vi "Library.GetMemberVIs.vi"(8 "error in (no error)":errorcluster, 11 "Library Reference":refnum<vi>) -> (0 "error out":errorcluster, 1 "Item Type":string[](array[string]), 2 "Member VI References":refnum<vi>[](array[refnum]), 3 "Library Reference (dup)":refnum<vi>)   [LabVIEW 2011]
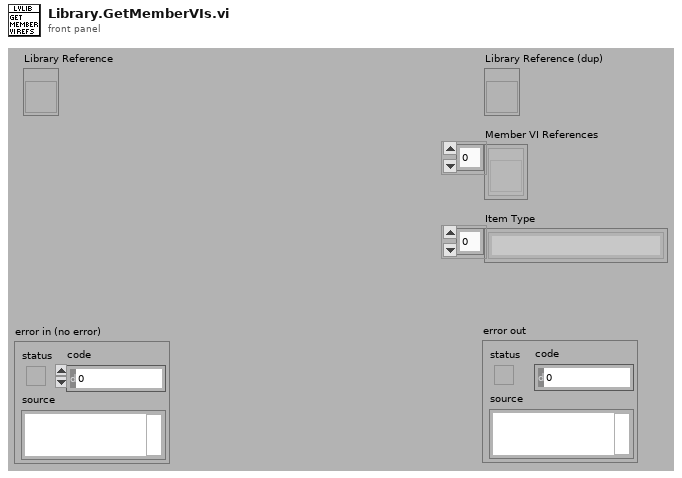
[diagram p1: front panel]
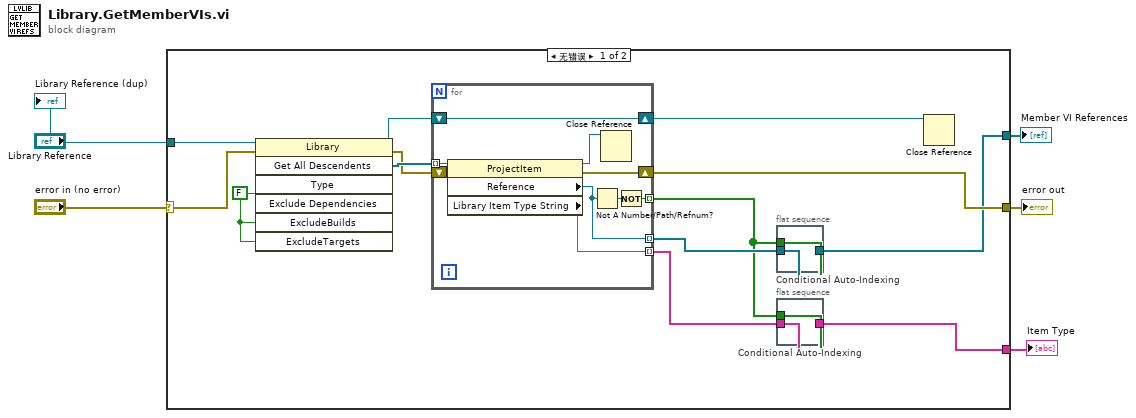
[diagram p0: block diagram]
diagram:
  n1 = case shown="无错误" "error in (no error)" {
    selector: "error in (no error)" -> [w13 w56]
    tunnel: [w10 _] -> w5
    tunnel: [w14 w56] -> w4
    tunnel: "Library Reference" -> [w6 _]
    tunnel: [w7 _] -> w1
    frame No Error {
      w12 = FALSE ("ExcludeDependencies")
      n2 = invoke class="Library" method="Get All Descendents"(reference=w6, error in=w13, "Exclude Dependencies"=w12, "ExcludeBuilds"=w12, "ExcludeTargets"=w12) -> (reference out=w16:refnum<vi>, error out=w17:errorcluster, "All Descendents"=w18:refnum<vi>[])  [unwired: 2 in, 4 out]
      n3 = for {
        tunnel: w18 -> [w55] mode=indexing
        tunnel: [w53] -> w9 mode=indexing
        tunnel: [w52] -> w11 mode=indexing
        shift-right: [w51] -> w14
        shift-left: w17 -> [w50]
        shift-right: [w48] -> w15
        shift-left: w16 -> [w48]
        tunnel: [w47] -> w8 mode=indexing
        n4 = property class="ProjectItem"(reference=w55, error in=w50) -> (reference out=w49:refnum<vi>, error out=w51:errorcluster, "Reference"=w52:refnum<vi>, "Library Item Type String"=w47:string)
        n5 = Not A Number/Path/Refnum?(number/path/refnum=w52) -> (NaN/Path/Refnum?=w54:bool)
        n6 = Close Reference(reference=w49) -> ()  [unwired: 1 in, 1 out]
        n7 = Not(x=w54) -> (.not. x?=w53:bool)
      }
      n8 = flat-sequence "Conditional Auto-Indexing" {
        tunnel: w9 -> [w35]
        tunnel: w11 -> [w34]
        tunnel: [w33] -> w10
        frame #0 {
          n9 = Boolean To (0,1)(Boolean=w35) -> (0, 1=w38:i16[])
          n10 = To Unsigned Long Integer(number=w38) -> (unsigned 32bit integer=w39:u32[])
          n11 = Add Array Elements(numeric array=w39) -> (sum=w37:u32)
          n12 = for {
            N: w37 -> [_]
            tunnel: w34 -> [w42]
            tunnel: w35 -> [w46]
            shift-right: [w43] -> _
            shift-left: -1 ("start index (0)") -> [w44]
            tunnel: [w41] -> w33 mode=indexing
            # "index out that element"
            # "Find the next element to keep"
            n13 = Increment(x=w44) -> (x+1=w40:i32)
            n14 = Search 1D Array(1D array=w46, element=TRUE, start index (0)=w40) -> (index of element=w43:i32)
            n15 = Index Array(array=w42, index=w43) -> (element=w41:refnum<vi>)
          }
        }
      }
      n16 = flat-sequence "Conditional Auto-Indexing" {
        tunnel: w9 -> [w21]
        tunnel: w8 -> [w20]
        tunnel: [w19] -> w7
        frame #0 {
          n17 = Boolean To (0,1)(Boolean=w21) -> (0, 1=w24:i16[])
          n18 = To Unsigned Long Integer(number=w24) -> (unsigned 32bit integer=w25:u32[])
          n19 = Add Array Elements(numeric array=w25) -> (sum=w23:u32)
          n20 = for {
            N: w23 -> [_]
            tunnel: w20 -> [w28]
            tunnel: w21 -> [w32]
            shift-right: [w29] -> _
            shift-left: -1 ("start index (0)") -> [w30]
            tunnel: [w27] -> w19 mode=indexing
            # "index out that element"
            # "Find the next element to keep"
            n21 = Increment(x=w30) -> (x+1=w26:i32)
            n22 = Search 1D Array(1D array=w32, element=TRUE, start index (0)=w26) -> (index of element=w29:i32)
            n23 = Index Array(array=w28, index=w29) -> (element=w27:string)
          }
        }
      }
      n24 = Close Reference(reference=w15) -> ()  [unwired: 1 in, 1 out]
    }
    frame Error {
    }
  }
  "Member VI References" <- w5
  "error out" <- w4
  "Item Type" <- w1
  "Library Reference (dup)" <- "Library Reference"
